vi "update pmt watchlist.vi"(4 "Watched Channels":path=path "C:/Users/User/Documents/Logs/PMT_watchlist.csv", 6 "Channels in Group00":T1[](array[typedef]) {"Card.Channel" format="%.2f"}, 8 "error in":errorcluster, 9 "Value":variant, 11 "Set Card.Channel":T1={" Card.Channel"=1.12, "Crate"=0} {"Card.Channel" format="%.2f"}) -> (0 "error out":errorcluster)   [LabVIEW 2018]
uses:
  channel.ctl
  <vilib>/Utility/file.llb/Read Delimited Spreadsheet (string).vi
  CAEN globals.vi
  <vilib>/Utility/file.llb/Write Delimited Spreadsheet (string).vi
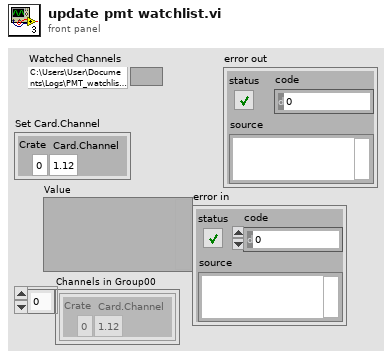
[diagram p1: front panel]
types:
  T1 = typedef "channel.ctl" = cluster{" Card.Channel":dbl, "Crate":i32}
  T2 = typedef "channel_cluster.ctl" = cluster{"Channel Name":string, "Crate":i32, "Card Type":string, "Card":i32, "Channel":i32, "Status Icon":picture, "Vmon (V)":dbl, "Vset (V)":dbl, "Imon (A)":dbl, "Iset (A)":dbl, "Timestamp":string, "ON/OFF":bool, "Status":string, "Vswmax (V)":dbl, "Flag":bool, "Vfile (V)":dbl, "Error Logged":bool[]}
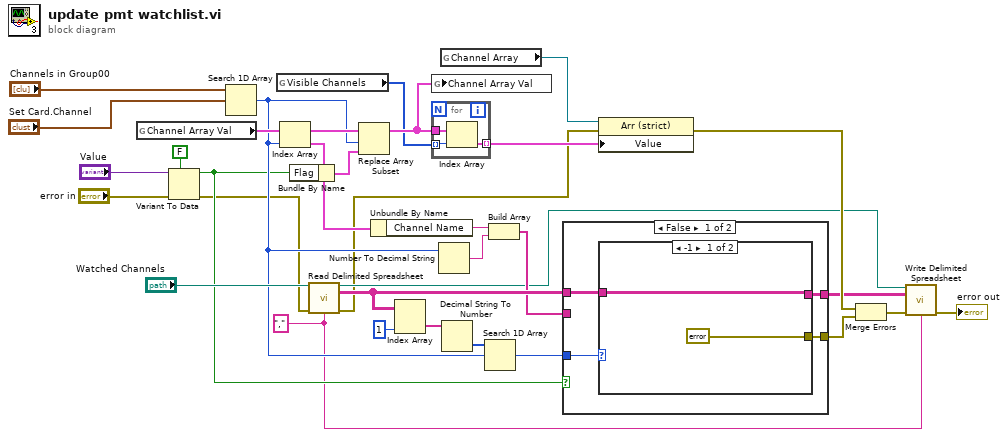
[diagram p0: block diagram]
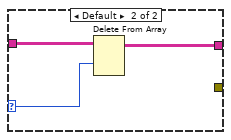
[diagram p2: hidden frame]
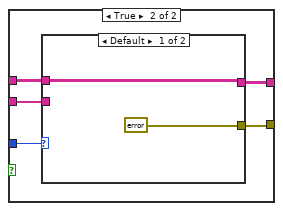
[diagram p3: hidden frame]
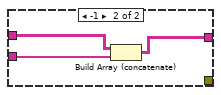
[diagram p4: hidden frame]
diagram:
  w5 = "," ("delimiter (\\t)")
  n1 = global read "CAEN globals.vi" "Channel Array Val"() -> (w29:T2[])
  n2 = Variant To Data(error in="error in", type=FALSE ("Set channel property"), Variant="Value") -> (data=w13:bool, error out=w2:errorcluster)
  n3 = Search 1D Array(1D array="Channels in Group00", element="Set Card.Channel") -> (index of element=w15:i32)  [unwired: 1 in]
  n4 = global read "CAEN globals.vi" "Visible Channels"() -> (w30:i32[])
  n5 = Index Array(array=w29, index=w15) -> (element=w21:T2)
  n6 = Bundle By Name(cluster=w21, "Flag"=w13) -> (w26:T2)
  n7 = call-poly <vilib>:"Read Delimited Spreadsheet.vi"("file path (dialog if empty)"="Watched Channels", "error in (no error)"=w2, "delimiter (\\t)"=w5) -> ("new file path (Not A Path if cancelled)"=w9:path, "all rows"=w14:string[][], "error out"=w1:errorcluster)  [unwired: 7 in, 3 out]
  n8 = Replace Array Subset(array=w29, new element=w26, index=w15) -> (w31:T2[])
  n9 = Unbundle By Name(w21) -> ("Channel Name"=w20:string)
  n10 = Index Array(array=w14, index (col)=1 ("disabled index (col)")) -> (element=w17:string[])  [unwired: 1 in]
  n11 = global write "CAEN globals.vi" "Channel Array Val"(w31) -> ()
  n12 = for {
    tunnel: w30 -> [w34] mode=indexing
    tunnel: w31 -> [w35]
    tunnel: [w33] -> w32 mode=indexing
    n13 = Index Array(array=w35, index=w34) -> (element=w33:T2)
  }
  n14 = Number To Decimal String(number=w15) -> (decimal integer string=w19:string)  [unwired: 1 in]
  n15 = global read "CAEN globals.vi" "Channel Array"() -> (w23:refnum<vi>)
  n16 = Decimal String To Number(string=w17) -> (number=w16:i32[])  [unwired: 2 in, 1 out]
  n17 = Search 1D Array(1D array=w16, element=w15) -> (index of element=w12:i32)  [unwired: 1 in]
  n18 = Build Array(w20, w19) -> (w11:string[])
  n19 = case shown="False" w13 {
    tunnel: w14 -> [w39 w49]
    tunnel: w12 -> [w37 w48]
    tunnel: [w38 w45] -> w8
    tunnel: [w36 w47] -> w7
    tunnel: w11 -> [_ w46]
    frame False {
      n20 = case shown="-1" w37 {
        selector: w37 -> [_ w42]
        tunnel: w39 -> [w40 w44]
        tunnel: [w40 w43] -> w38
        tunnel: [errorcluster {"status"=TRUE, "code"=0, "source"="Attempt to remove flag from unflagged channel!"} ("error out") _] -> w36
        frame -1 {
        }
        frame Default {
          n21 = Delete From Array(array=w44, index (row)=w42) -> (array with subset deleted=w43:string[][])  [unwired: 2 in, 1 out]
        }
      }
    }
    frame True {
      n22 = case shown="Default" w48 {
        tunnel: w49 -> [w50 w54]
        tunnel: [errorcluster {"status"=TRUE, "code"=0, "source"="Attempt to flag already flagged channel!"} ("error out") _] -> w47
        tunnel: w46 -> [_ w53]
        tunnel: [w50 w52] -> w45
        frame Default {
        }
        frame -1 {
          n23 = Build Array (concatenate)(w54, w53) -> (w52:string[][])
        }
      }
    }
  }
  n24 = property class="Arr (strict)"(reference=w23, error in=w1, "Value"=w32) -> (error out=w10:errorcluster)  [unwired: 1 out]
  n25 = Merge Errors(w10, w7) -> (w6:errorcluster)
  n26 = call-poly <vilib>:"Write Delimited Spreadsheet.vi"("file path (dialog if empty)"=w9, "2D data"=w8, "error in (no error)"=w6, "delimiter (\\t)"=w5) -> ("error out"=→"error out":errorcluster)  [unwired: 10 in, 1 out]
